vi "test_OpticalLevel_rt.vi"() -> ()   [LabVIEW 2020]
uses:
  <vilib>/FPGAPlugInAG/cRIO-9049/niLvFpga_Open_cRIO-9049.vi
  <vilib>/Utility/error.llb/Error Cluster From Error Code.vi
  <vilib>/rvi/errors/niLvFpgaAdjustHostInterfaceError.vi
  <vilib>/FPGAPlugInAG/cRIO-9049/niLvFpga_Run_cRIO-9049.vi
  <vilib>/FPGAPlugInAG/cRIO-9049/niLvFpga_Close_cRIO-9049.vi
  <vilib>/rvi/interface/nirviOpenFPGA/nirviOpenFPGA.xnode
  FPGA Bitfiles/testopticallevel_FPGATarget_testOpticalLevel_QDmyqR17CYI.lvbitx
  test_OpticalLevel_fpga.vi
  <vilib>/rvi/interface/nirviReadWriteControl/nirviReadWriteControl.xnode
  <vilib>/rvi/interface/nirviMethod/nirviMethod.xnode
  <vilib>/rvi/interface/nirviCloseFPGA/nirviCloseFPGA.xnode
  NiFpgaLv.dll
  <vilib>/FPGAPlugInAG/cRIO-9049/niLvFpga_ReadFifo_cRIO-9049.vi
  <vilib>/rvi/errors/niLvFpgaMergeErrorWithErrorCode.vi
panel:
  out "XY Graph":cluster{sgl[], sgl[]}(graph)
  out "0":sgl[](array[numeric])
  out "Time string":string="05/19/2021 13:25:56.954636"
  out "Filename Out":path=path "/home/lvuser/natinst/LABVIEWData/SCI_21-05-19_1322.lvm"
  in  "decimation":i16=25
  in  "Enable":bool
  out "Saving Data":bool
  out "Dx_norm":sgl[](graph)
  out "Dy_norm":sgl[](graph)
  out "Elements Remaining":u32
  out "Sum":sgl[](graph)
  in  "Number of Elements":u32=400
  in  "stop":bool
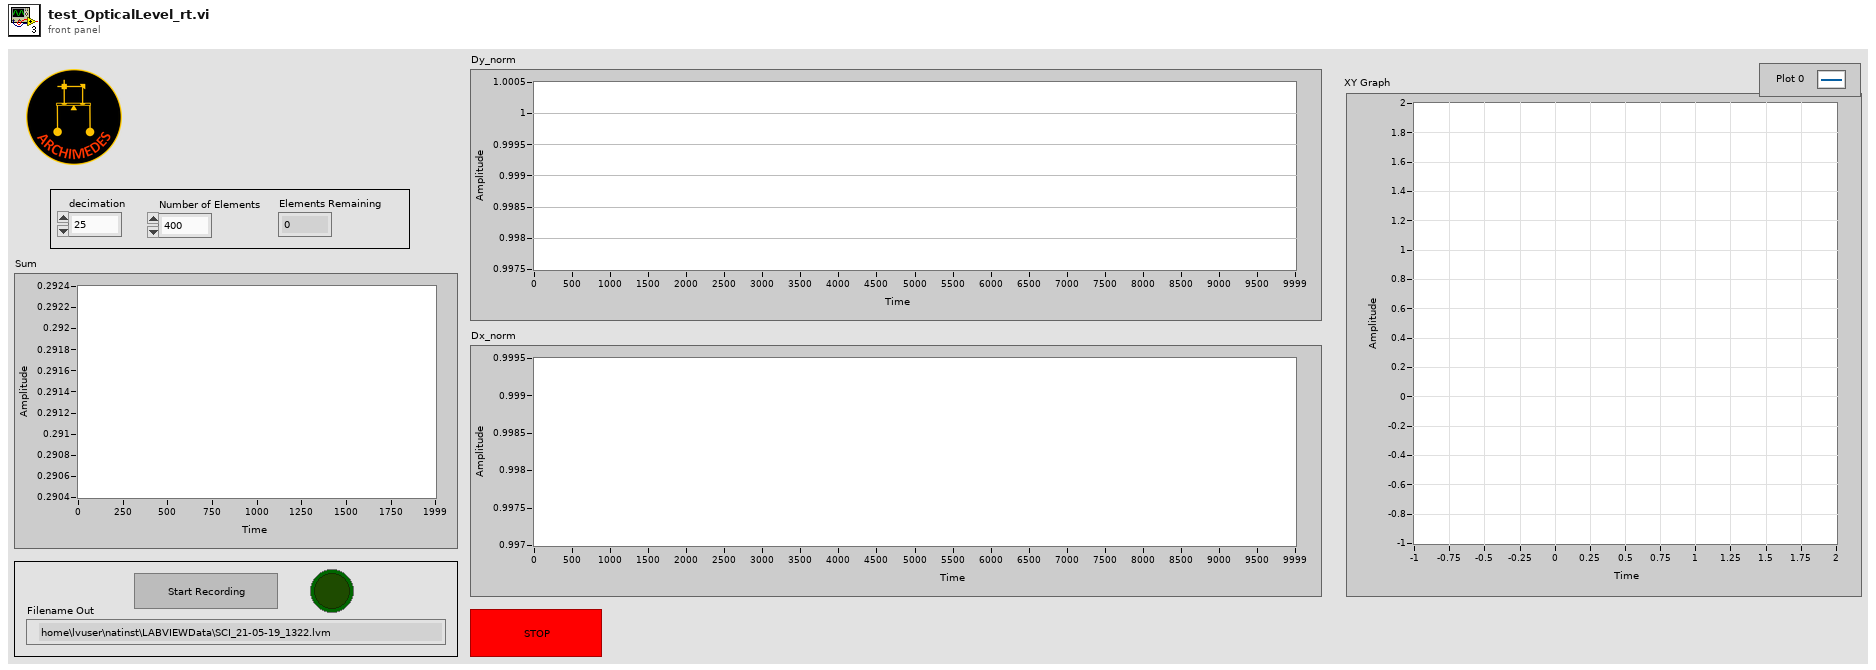
[diagram p1: front panel]
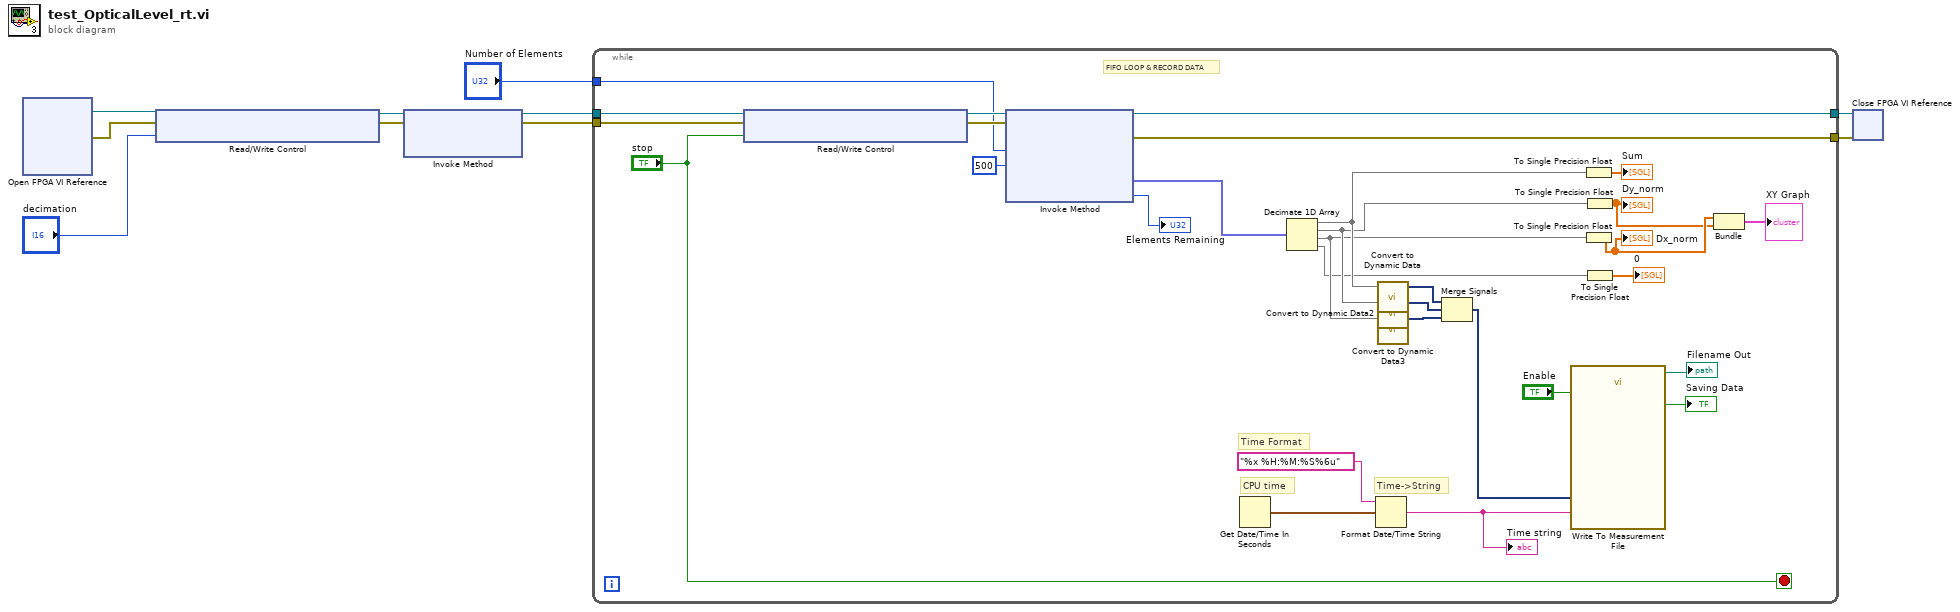
[diagram p0: block diagram]
diagram:
  n1 = xnode "Open FPGA VI Reference"() -> ("FPGA VI Reference Out"=w6:refnum<k20>, "error out"=w5:errorcluster)  [unwired: 2 in]
  n2 = xnode "Read/Write Control"("FPGA VI Reference In"=w6, "error in"=w5, "decimation"="decimation") -> ("FPGA VI Reference Out"=w3:refnum<k20>, "error out"=w2:errorcluster)
  n3 = xnode "Invoke Method"("FPGA VI Reference In"=w3, "error in"=w2) -> ("FPGA VI Reference Out"=w9:refnum<k20>, "error out"=w10:errorcluster)  [unwired: 1 in]
  n4 = while {
    tunnel: w10 -> [w40]
    tunnel: w9 -> [w39]
    tunnel: [w38] -> w8
    tunnel: [w37] -> w4
    tunnel: "Number of Elements" -> [w34]
    stop <- "stop" stop-if-true
    # "FIFO LOOP & RECORD DATA"
    # "Time->String"
    # "CPU time"
    # "Time Format"
    n5 = xnode "Read/Write Control"("FPGA VI Reference In"=w39, "error in"=w40, "stop"="stop") -> ("FPGA VI Reference Out"=w36:refnum<k20>, "error out"=w35:errorcluster)
    n6 = xnode "Invoke Method"("FPGA VI Reference In"=w36, "error in"=w35, "Number of Elements"=w34, "Timeout (ms)"=500) -> ("FPGA VI Reference Out"=w38:refnum<k20>, "error out"=w37:errorcluster, "Data"=w31:fxp<+/-,64,20>[], "Elements Remaining"=→"Elements Remaining":u32)
    n7 = Get Date/Time In Seconds() -> (seconds since 1Jan1904=w24:timestamp)
    n8 = Decimate 1D Array(w31) -> (w18:fxp<+/-,64,20>[], w17:fxp<+/-,64,20>[], w16:fxp<+/-,64,20>[], w15:fxp<+/-,64,20>[])
    n9 = Format Date/Time String(time format string (%c)="%x %H:%M:%S%6u", seconds (now)=w24) -> (date/time string=w19:string)  [unwired: 1 in]
    "Time string" <- w19
    n10 = call "Convert to Dynamic Data"("Array"=w18) -> ("Dynamic Data Type"=w30:dynamicdata)  [unwired: 3 in]
    n11 = call "Convert to Dynamic Data2"("Array"=w17) -> ("Dynamic Data Type"=w29:dynamicdata)  [unwired: 3 in]
    n12 = call "Convert to Dynamic Data3"("Array"=w16) -> ("Dynamic Data Type"=w27:dynamicdata)  [unwired: 3 in]
    n13 = Merge Signals(w30, w29, w27) -> (w28:dynamicdata)
    n14 = call "Write To Measurement File"("Signals"=w28, "Enable"="Enable", "Comment"=w19) -> ("Filename Out"=→"Filename Out":path, "Saving Data"=→"Saving Data":bool)  [unwired: 14 in, 1 out]
    n15 = To Single Precision Float(number=w18) -> (single precision float=→"Sum":sgl[])
    n16 = To Single Precision Float(number=w16) -> (single precision float=w13:sgl[])
    "Dx_norm" <- w13
    n17 = To Single Precision Float(number=w17) -> (single precision float=w12:sgl[])
    "Dy_norm" <- w12
    n18 = To Single Precision Float(number=w15) -> (single precision float=→"0":sgl[])
    n19 = Bundle(w13, w12) -> (→"XY Graph":cluster{sgl[], sgl[]})  [unwired: 1 in]
  }
  n20 = xnode "Close FPGA VI Reference"("FPGA VI Reference In"=w8, "error in"=w4) -> ()  [unwired: 1 out]
